vi "Ping_Arduino.vi"(8 "error in (no error)":errorcluster, 10 "VISA resource name":refnum<visa-resource-name>, 11 "input cluster":T1) -> (0 "error IO":errorcluster, 2 "VISA resource name out":refnum<visa-resource-name>)   [LabVIEW 2019]
uses:
  Type_defs/REFERENCIAS_CONTROLES_INDICADORES.ctl
  <vilib>/Utility/error.llb/Error Cluster From Error Code.vi
  <vilib>/ErrorRing/Error Ring.xnode
panel:
  out "ARDUINO MESSAGES":string
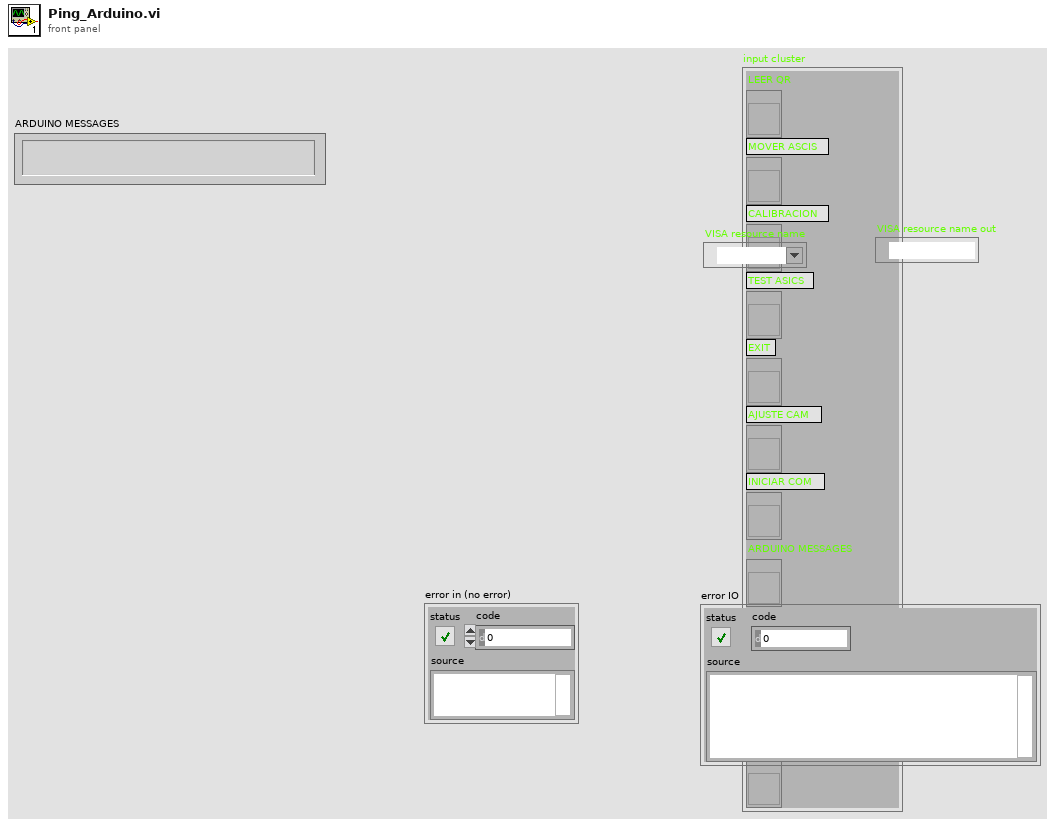
[diagram p1: front panel]
types:
  T1 = typedef "REFERENCIAS_CONTROLES_INDICADORES.ctl" = cluster{"LEER QR":refnum<vi>, "MOVER ASCIS":refnum<vi>, "CALIBRACION":refnum<vi>, "TEST ASICS":refnum<vi>, "EXIT":refnum<vi>, "AJUSTE CAM":refnum<vi>, "INICIAR COM":refnum<vi>, "ARDUINO MESSAGES":refnum<vi>, "LABVIEW MESSAGES":refnum<vi>, "DISPOSITIVO CONECTADO":refnum<vi>, "Config Estación":refnum<vi>}
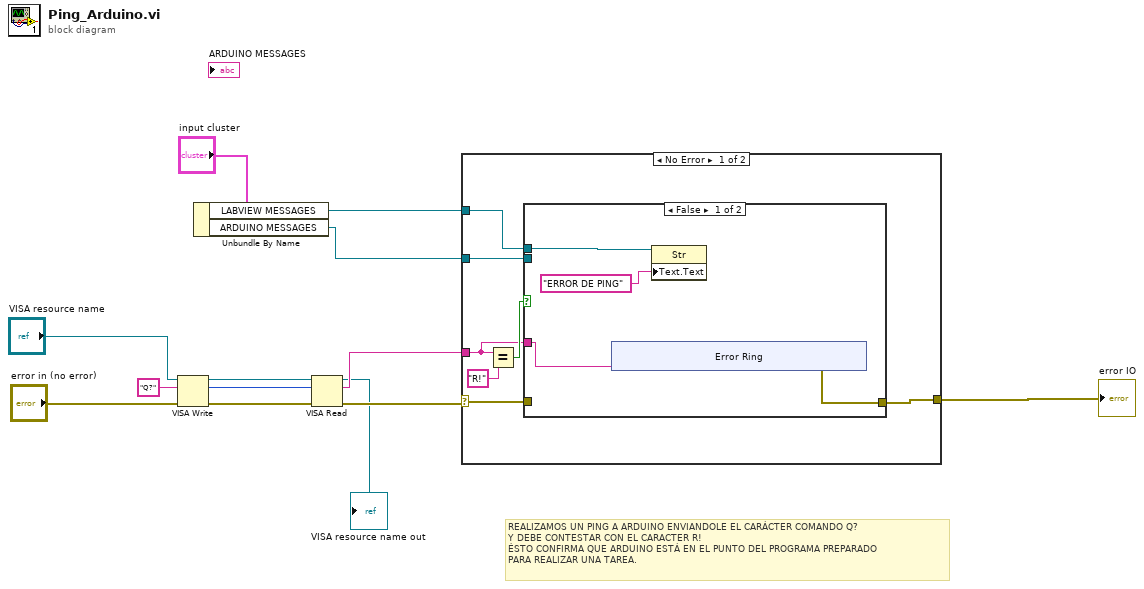
[diagram p0: block diagram]
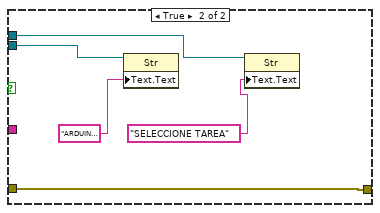
[diagram p2: hidden frame]
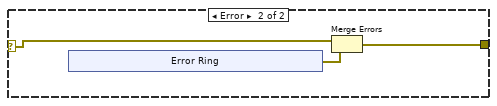
[diagram p3: hidden frame]
diagram:
  # "REALIZAMOS UN PING A ARDUINO ENVIANDOLE EL CARÁCTER COMANDO Q?\nY DEBE CONTESTAR CON EL CARACTER R!\nÉSTO CONFIRMA QUE ARDUINO ESTÁ EN EL PUNTO DEL PROGRAMA PREPARADO \nPARA REALIZAR UNA TAREA."
  n1 = VISA Write(VISA resource name="VISA resource name", write buffer="Q?", error in (no error)="error in (no error)") -> (VISA resource name out=w12:refnum<visa-resource-name>, return count=w3:u32, error out=w1:errorcluster)
  n2 = Unbundle By Name("input cluster") -> ("LABVIEW MESSAGES"=w10:refnum<vi>, "ARDUINO MESSAGES"=w9:refnum<vi>)
  n3 = VISA Read(VISA resource name=w12, byte count=w3, error in (no error)=w1) -> (VISA resource name out=→"VISA resource name out":refnum<visa-resource-name>, read buffer=w6:string, error out=w7:errorcluster)  [unwired: 1 out]
  n4 = case shown="No Error" w7 {
    selector: w7 -> [w15 w38]
    tunnel: [w20 w37] -> w4
    tunnel: w10 -> [w19 _]
    tunnel: w9 -> [w18 _]
    tunnel: w6 -> [w14 _]
    frame No Error {
      n5 = Equal?(x=w14, y="R!") -> (x = y?=w16:bool)
      n6 = case shown="False" w16 {
        tunnel: [w24 w32] -> w20
        tunnel: w19 -> [w23 w34]
        tunnel: w18 -> [_ w36]
        tunnel: w15 -> [_ w32]
        tunnel: w14 -> [w21 _]
        frame False {
          n7 = xnode "Error Ring"("parameter 0"=w21) -> ("error out"=w24:errorcluster)
          n8 = property class="Str"(reference=w23, "Text.Text"="ERROR DE PING" ("Text")) -> ()  [unwired: 1 in, 2 out]
        }
        frame True {
          n9 = property class="Str"(reference=w36, "Text.Text"="ARDUINO READY!" ("ARDUINO MESSAGES")) -> ()  [unwired: 1 in, 2 out]
          n10 = property class="Str"(reference=w34, "Text.Text"="SELECCIONE TAREA" ("Text")) -> ()  [unwired: 1 in, 2 out]
        }
      }
    }
    frame Error {
      n11 = xnode "Error Ring"() -> ("error out"=w39:errorcluster)
      n12 = Merge Errors(w38, w39) -> (w37:errorcluster)
    }
  }
  "error IO" <- w4
